vi "Facade.vi"(0 "Data In":T4, 2 "Display State In":T2, 3 "Container State":T3) -> (6 "Data Out":T4, 7 "Display State Out":T2, 8 "Action":T1)   [LabVIEW 2015, in "File.xctl"]
uses:
  File.xctl
  Data.vi
  Classes/Waveforms/File/File.lvclass
  <vilib>/_xctls/Container State.ctl
  State.vi
  <vilib>/_xctls/Action.ctl
  Classes/Waveforms/File/File.lvclass/File.ctl
  Classes/Waveforms/File/Read Filename.vi
  Classes/Waveforms/File/Write Filename.vi
  <vilib>/_xctls/XControlSupport.lvlib
panel:
  in  "Filename":path
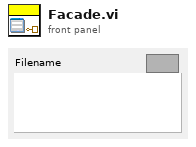
[diagram p1: front panel]
types:
  T1 = typedef "XControlSupport.lvlib/Action.ctl" = cluster{"Data Changed?":bool, "State Changed?":bool, "Action Name":string}
  T2 = typedef "File.xctl/State.vi" = cluster{"Numeric":dbl}
  T3 = typedef "XControlSupport.lvlib/Container State.ctl" = cluster{"Indicator?":bool, "Run Mode?":bool, " Refnum":refnum<vi>}
  T4 = typedef "File.xctl/Data.vi" = refnum<class "File.lvclass">
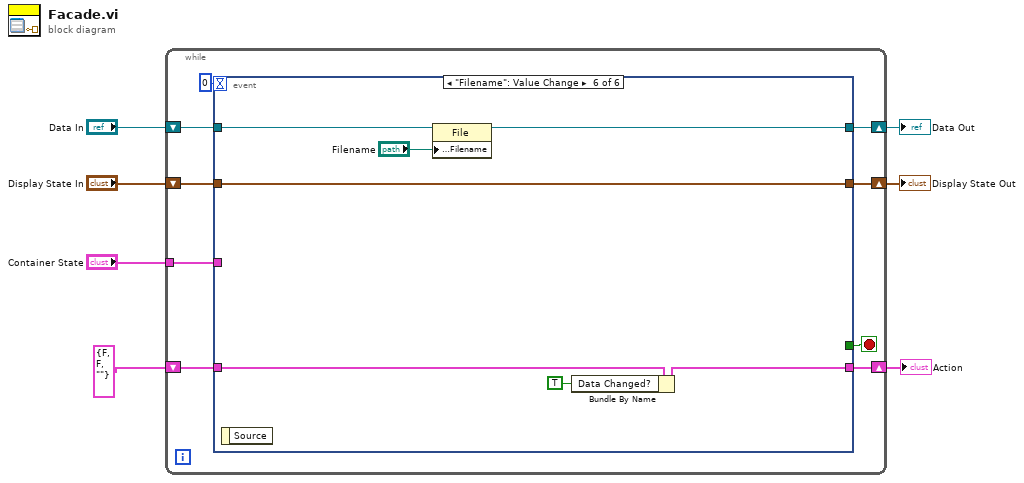
[diagram p0: block diagram]
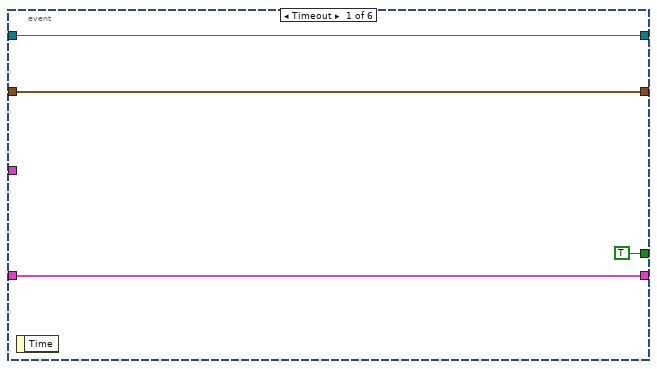
[diagram p2: hidden frame]
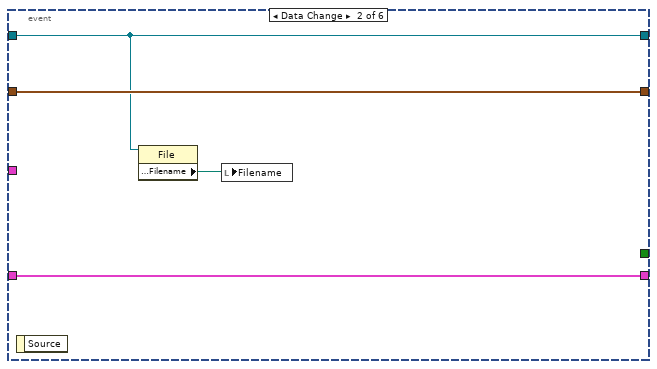
[diagram p3: hidden frame]
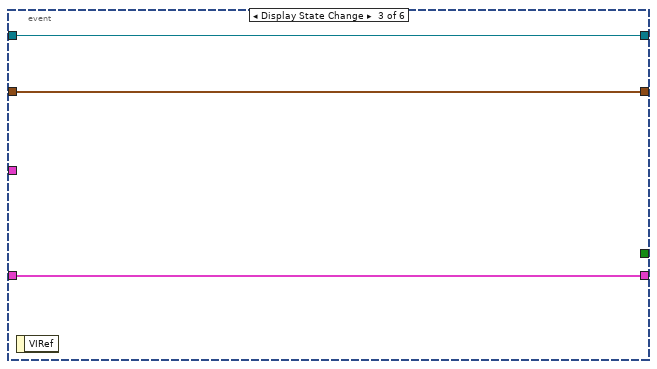
[diagram p4: hidden frame]
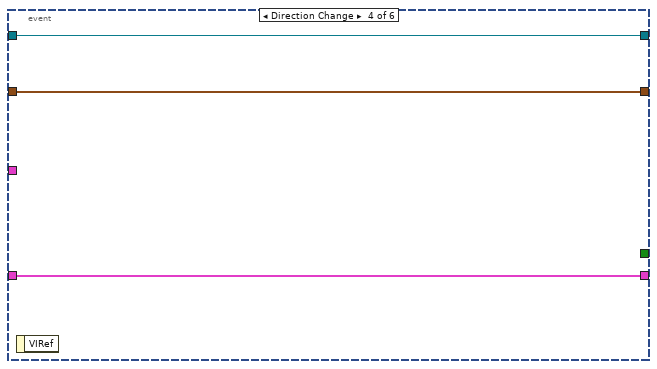
[diagram p5: hidden frame]
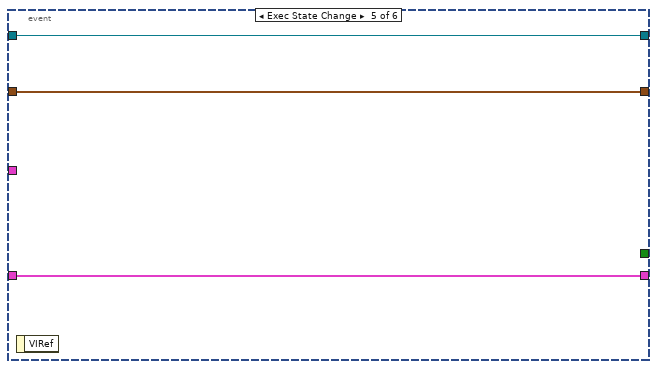
[diagram p6: hidden frame]
diagram:
  n1 = while {
    shift-right: [w15] -> w4
    shift-left: "Display State In" -> [w16]
    tunnel: "Container State" -> [w12]
    shift-right: [w10] -> w7
    shift-left: "Data In" -> [w11]
    shift-right: [w8] -> w2
    shift-left: T1 {"Data Changed?"=FALSE, "State Changed?"=FALSE, "Action Name"=""} ("Action") -> [w9]
    stop <- w14 stop-if-true
    n2 = event shown="[5] \"Filename\": Value Change" {
      selector: _ -> [_ _ _ _ _ _]
      dyn-events: _ -> [_ _ _ _ _ _]
      timeout: 0 -> [_ _ _ _ _ _]
      tunnel: w16 -> [w18 w24 w27 w30 w33 w40]
      tunnel: [w18 w24 w27 w30 w33 w40] -> w15
      tunnel: [TRUE _ _ _ _ _] -> w14
      tunnel: w12 -> [_ _ _ _ _ _]
      tunnel: w11 -> [w17 w22 w26 w29 w32 w39]
      tunnel: [w17 w22 w26 w29 w32 w37] -> w10
      tunnel: [w19 w23 w25 w28 w31 w35] -> w8
      tunnel: w9 -> [w19 w23 w25 w28 w31 w38]
      event Timeout {
        n3 = event-data() -> ()  [unwired: 1 in, 1 out]
      }
      event Data Change {
        n4 = event-data() -> ()  [unwired: 1 in, 1 out]
        n5 = property class="File"(reference=w22) -> ("Accessors:Filename"=w21:path)  [unwired: 1 in, 2 out]
        n6 = local write "Filename"(w21) -> ()
      }
      event Display State Change {
        n7 = event-data() -> ()  [unwired: 1 in, 1 out]
      }
      event Direction Change {
        n8 = event-data() -> ()  [unwired: 1 in, 1 out]
      }
      event Exec State Change {
        n9 = event-data() -> ()  [unwired: 1 in, 1 out]
      }
      event "Filename": Value Change {
        n10 = event-data() -> ()  [unwired: 1 in, 1 out]
        n11 = property class="File"(reference=w39, "Accessors:Filename"="Filename") -> (reference out=w37:T4)  [unwired: 1 in, 1 out]
        n12 = Bundle By Name(cluster=w38, "Data Changed?"=TRUE) -> (w35:T1)
      }
    }
  }
  "Display State Out" <- w4
  "Data Out" <- w7
  "Action" <- w2
